vi "FisherPaykel Friction Profile.vi"(7 "Debug":bool, 8 "Error In":errorcluster, 9 "Move With Friction Test Profile":T1, 10 "Main Command":T2=">GF", 11 "VISA Refnum in":refnum<visa-resource-name>) -> (0 "Error Out":errorcluster, 2 "Command (Debug)":string, 3 "VISA Refnum out":refnum<visa-resource-name>)   [LabVIEW 2016]
uses:
  Type Definitions/Fisher Paykel Main Command.ctl
  Type Definitions/Fisher Paykel Friction Profile.ctl
panel:
  # "Start Speed > End Speed"
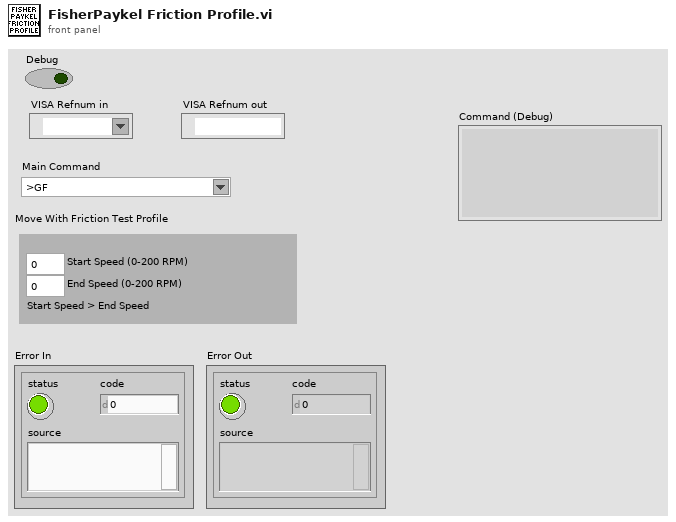
[diagram p1: front panel]
types:
  T1 = typedef "Fisher Paykel Friction Profile.ctl" = cluster{"Start Speed (0-200 RPM)":u16, "End Speed (0-200 RPM)":u16}
  T2 = typedef "Fisher Paykel Main Command.ctl" = string
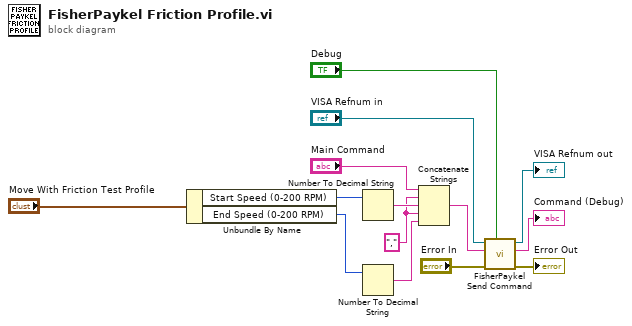
[diagram p0: block diagram]
diagram:
  w2 = ","
  n1 = Unbundle By Name("Move With Friction Test Profile") -> ("Start Speed (0-200 RPM)"=w6:u16, "End Speed (0-200 RPM)"=w5:u16)
  n2 = Number To Decimal String(number=w6) -> (decimal integer string=w4:string)  [unwired: 1 in]
  n3 = Number To Decimal String(number=w5) -> (decimal integer string=w3:string)  [unwired: 1 in]
  n4 = Concatenate Strings("Main Command", w2, w4, w2, w3) -> (w13:string)
  n5 = call "FisherPaykel Send Command.vi"("Debug"="Debug", "error in (no error)"="Error In", "Send Command"=w13, "VISA Refnum in"="VISA Refnum in") -> ("error out"=→"Error Out":errorcluster, "Command (Debug)"=→"Command (Debug)":string, "VISA Refnum out"=→"VISA Refnum out":refnum<visa-resource-name>)  [unwired: 5 in]
